vi "VoltChnSet.vi"(4 "相位输入":sgl[](array[numeric]), 5 "HIFU":bool, 6 "error in (no error)":errorcluster, 7 "chn num":i16=110, 8 "SeqNum":u32, 9 "connection ID in":refnum<k5>) -> (0 "error out":errorcluster, 1 "SeqOUT":u32, 2 "OK?":bool, 3 "connection ID out":refnum<k5>)   [LabVIEW 2016]
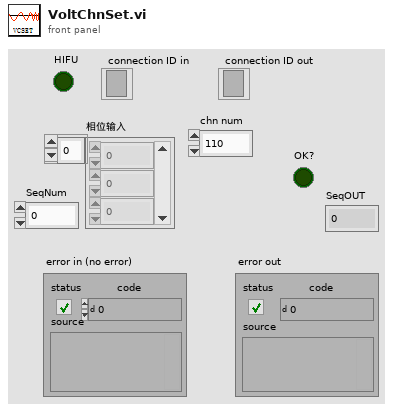
[diagram p1: front panel]
types:
  T1 = enum8{"SET_VOLT", "SET_CHANNEL_VOLT", "SET_PHASE", "START_HEAT", "STOP_HEAT", "CHANNEL_CTRL_SINGLE", "CHANNEL_CTRL_ALL", "READ_VOLT_SET", "READ_VOLT_SET_RSP", "READ_CURRENT_VOLT", "READ_CURRENT_VOLT_RSP", "READ_PHASE", "READ_PHASE_RSP", "READ_HEATTIME_LEFT", "READ_HEATTIME_LEFT_RSP", "EXEC_RSP"}
  T2 = enum8{"SET_VOLT", "SET_CHENNEL_VOLT", "SET_PHASE", "START_HEAT", "STOP_HEAT", "CHANNEL_CTRL_SINGLE", "CHANNEL_CTRL_ALL", "READ_VOLT_SET", "READ_VOLT_SET_RSP", "READ_CURRENT_VOLT", "READ_CURRENT_VOLT_RSP", "READ_PHASE", "READ_PHASE_RSP", "READ_HEATTIME_LEFT", "READ_HEATTIME_LEFT_RSP", "EXEC_RSP"}
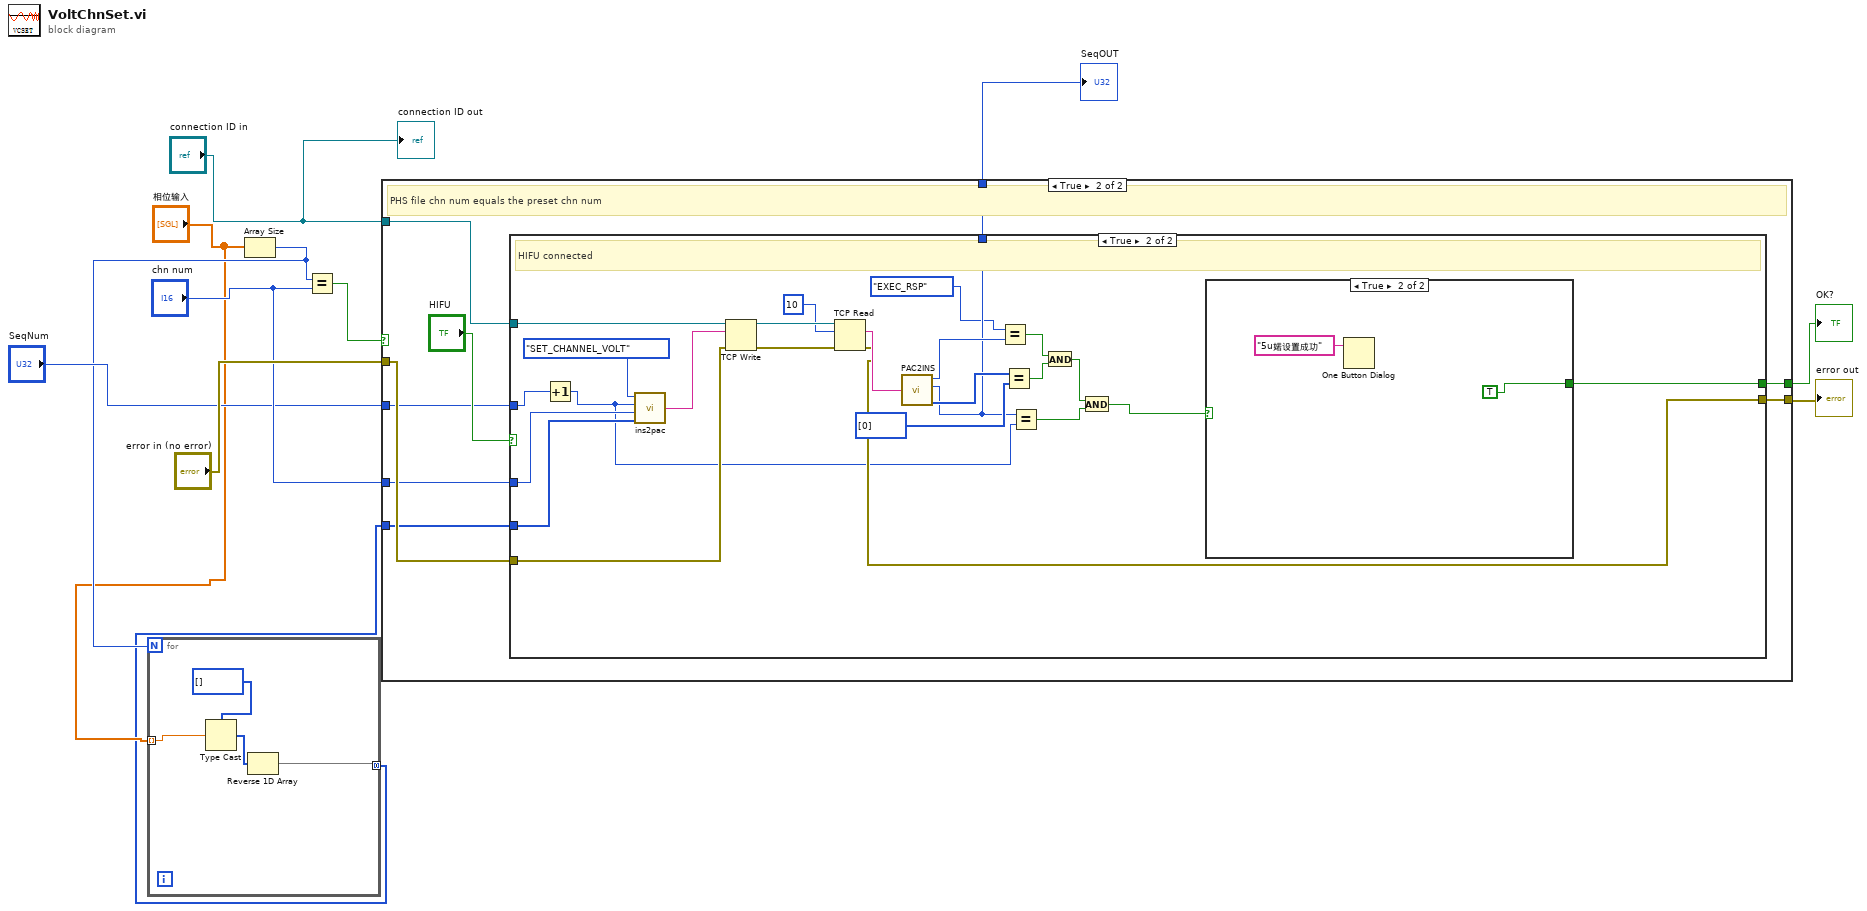
[diagram p0: block diagram]
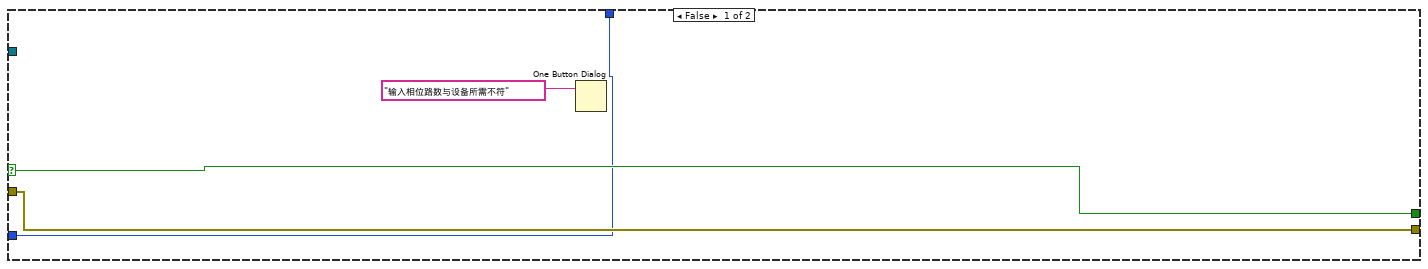
[diagram p2: hidden frame]
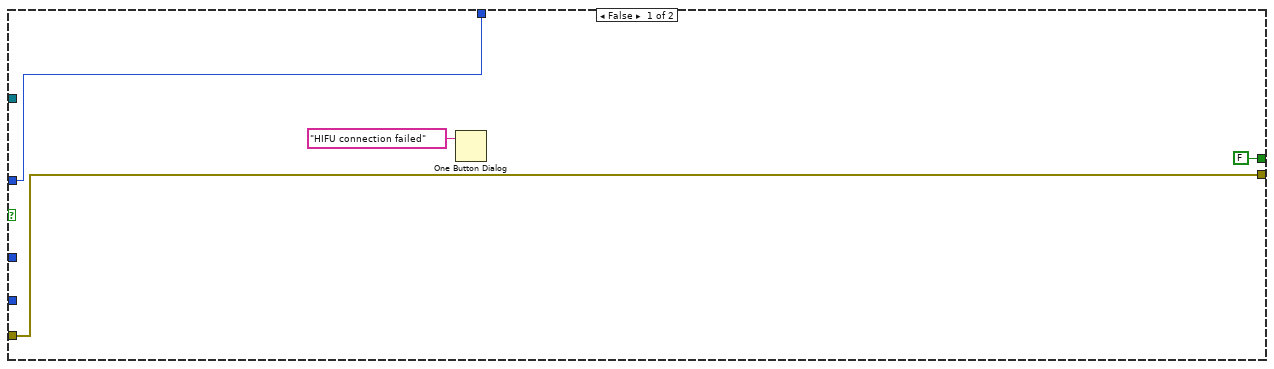
[diagram p3: hidden frame]
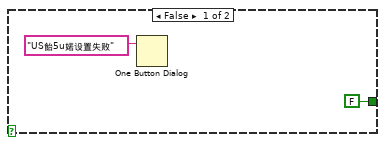
[diagram p4: hidden frame]
diagram:
  n1 = Array Size(array="相位输入") -> (size(s)=w3:i32)
  n2 = for {
    N: w3 -> [_]
    tunnel: "相位输入" -> [w15] mode=indexing
    tunnel: [w12] -> w1 mode=concatenating
    n3 = Type Cast(type=u8[] [], x=w15) -> (*(type *) &x=w13:u8[])
    n4 = Reverse 1D Array(array=w13) -> (reversed array=w12:u8[])
  }
  n5 = Equal?(x=w3, y="chn num") -> (x = y?=w11:bool)
  n6 = case shown="True" w11 {
    selector: w11 -> [w18 _]
    tunnel: "error in (no error)" -> [w17 w27]
    tunnel: [w18 w21] -> w9
    tunnel: [w17 w26] -> w8
    tunnel: "chn num" -> [_ w25]
    tunnel: w1 -> [_ w24]
    tunnel: "SeqNum" -> [w16 w23]
    tunnel: "connection ID in" -> [_ w22]
    tunnel: [w16 w20] -> w4
    frame False {
      n7 = One Button Dialog(message="输入相位路数与设备所需不符") -> ()  [unwired: 1 in, 1 out]
    }
    frame True {
      # "PHS file chn num equals the preset chn num"
      n8 = case shown="True" "HIFU" {
        tunnel: w27 -> [w31 w53]
        tunnel: [w31 w37] -> w26
        tunnel: w25 -> [_ w52]
        tunnel: w24 -> [_ w51]
        tunnel: w23 -> [w29 w36]
        tunnel: w22 -> [_ w55]
        tunnel: [FALSE w38] -> w21
        tunnel: [w29 w34] -> w20
        frame False {
          n9 = One Button Dialog(message="HIFU connection failed") -> ()  [unwired: 1 in, 1 out]
        }
        frame True {
          # "HIFU connected"
          n10 = Increment(x=w36) -> (x+1=w35:u32)
          n11 = call "ins2pac.vi"("BODY"=w51, "chn num"=w52, "SEQUENCE"=w35, "TYPE"=T1."SET_CHANNEL_VOLT") -> ("PACKET"=w54:string)
          n12 = TCP Write(connection ID=w55, data in=w54, error in (no error)=w53) -> (connection ID out=w49:refnum<k5>, error out=w50:errorcluster)  [unwired: 1 in, 1 out]
          n13 = TCP Read(connection ID=w49, bytes to read=10, error in (no error)=w50) -> (data out=w47:string, error out=w37:errorcluster)  [unwired: 2 in, 1 out]
          n14 = call "PAC2INS.vi"("PACKET"=w47) -> ("TYPE"=w46:T2, "SEQUENCE"=w34:u32, "BODY"=w44:u8[])  [unwired: 1 out]
          n15 = Equal?(x=T1."EXEC_RSP" ("TYPE"), y=w46) -> (x = y?=w43:bool)
          n16 = Equal?(x=w44, y=i32[] [0]) -> (x = y?=w42:bool)
          n17 = Equal?(x=w34, y=w35) -> (x = y?=w40:bool)
          n18 = And(x=w43, y=w42) -> (x .and. y?=w41:bool)
          n19 = And(x=w41, y=w40) -> (x .and. y?=w39:bool)
          n20 = case shown="True" w39 {
            tunnel: [FALSE TRUE] -> w38
            frame False {
              n21 = One Button Dialog(message="US飴5u婼设置失败") -> ()  [unwired: 1 in, 1 out]
            }
            frame True {
              n22 = One Button Dialog(message="5u婼设置成功") -> ()  [unwired: 1 in, 1 out]
            }
          }
        }
      }
    }
  }
  "error out" <- w8
  "OK?" <- w9
  "SeqOUT" <- w4
  "connection ID out" <- "connection ID in"
